vi "tcp发送-main.vi"(0 "服务器网络地址":string="127.0.0.1", 5 "原文件路径（使用对话框）":path=path "C:/Users/Administrator.2W964MZOGI5HE3B/Desktop/labview图片/105256rhad11pc5553vz5e.png", 7 "远程端口或服务名称":u16=6314) -> (4 "运行指示灯":bool=TRUE, 6 "已传百分比":string)   [LabVIEW 2016, in "数据传输系统.lvlib" / "自动更新.lvlib" / "TCP文件传输系统.lvlib" / "TCP发送文件.lvlib"]
panel:
  out "数值":i32
  in  "分帧数(兆)":i64=2
  out "已发帧数":i32
  in  "分一包（兆）":i64=40
  out "侦数":i32
  out "在发第几次":i32
  out "共发送次数":string
  out "网络灯":bool
  in  "停止":bool
  out "错误输出 2":errorcluster caption="错误输出"
  out "错误输出":errorcluster
  out "文件名称":string
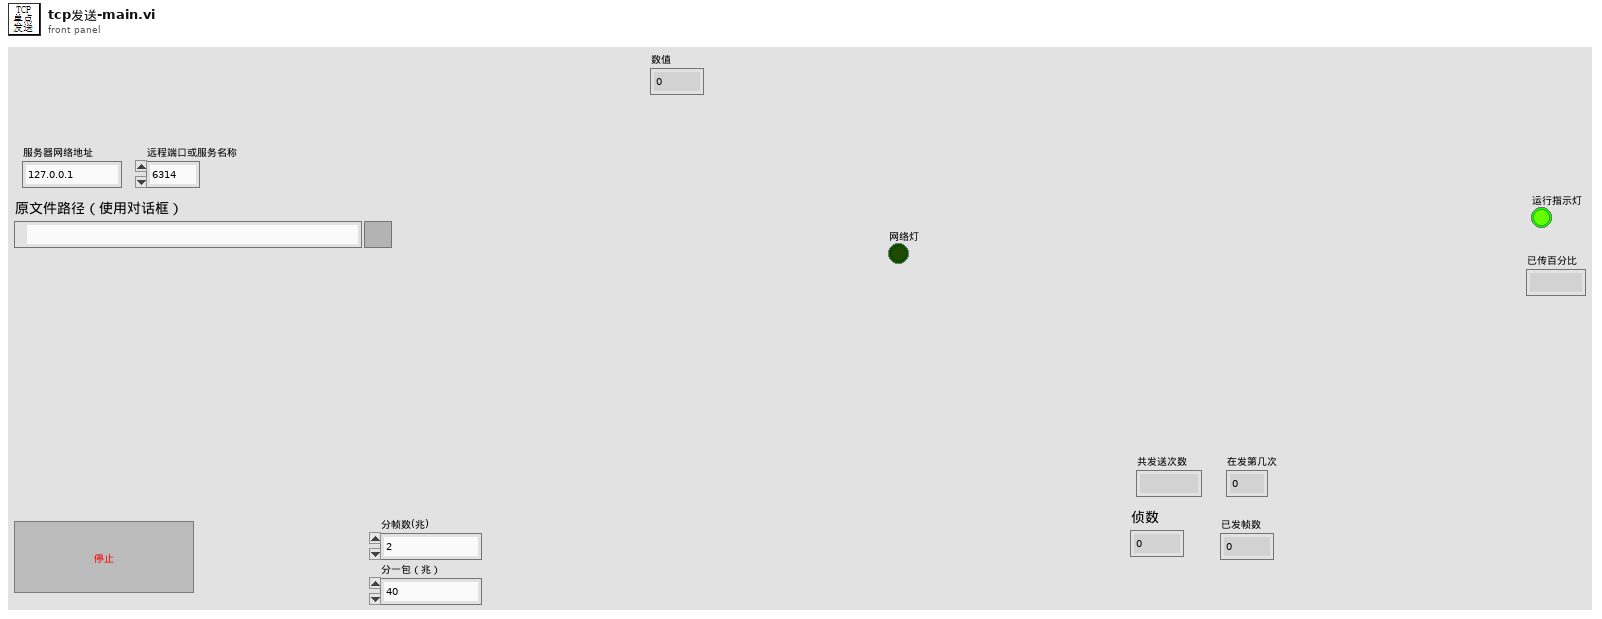
[diagram p1: front panel]
types:
  T1 = enum16{"open", "replace", "create", "open or create", "replace or create", "replace or create with confirmation"}
  T2 = cluster{"网络灯":bool, "发送中":bool, "已发送百分比":u8, "发送成功次数":dbl, "当前步骤":enum16{"readfile", "init", "sendhead", "sendcontent", "sendsuccess", "over"}, "文件名":string, "error out":errorcluster}
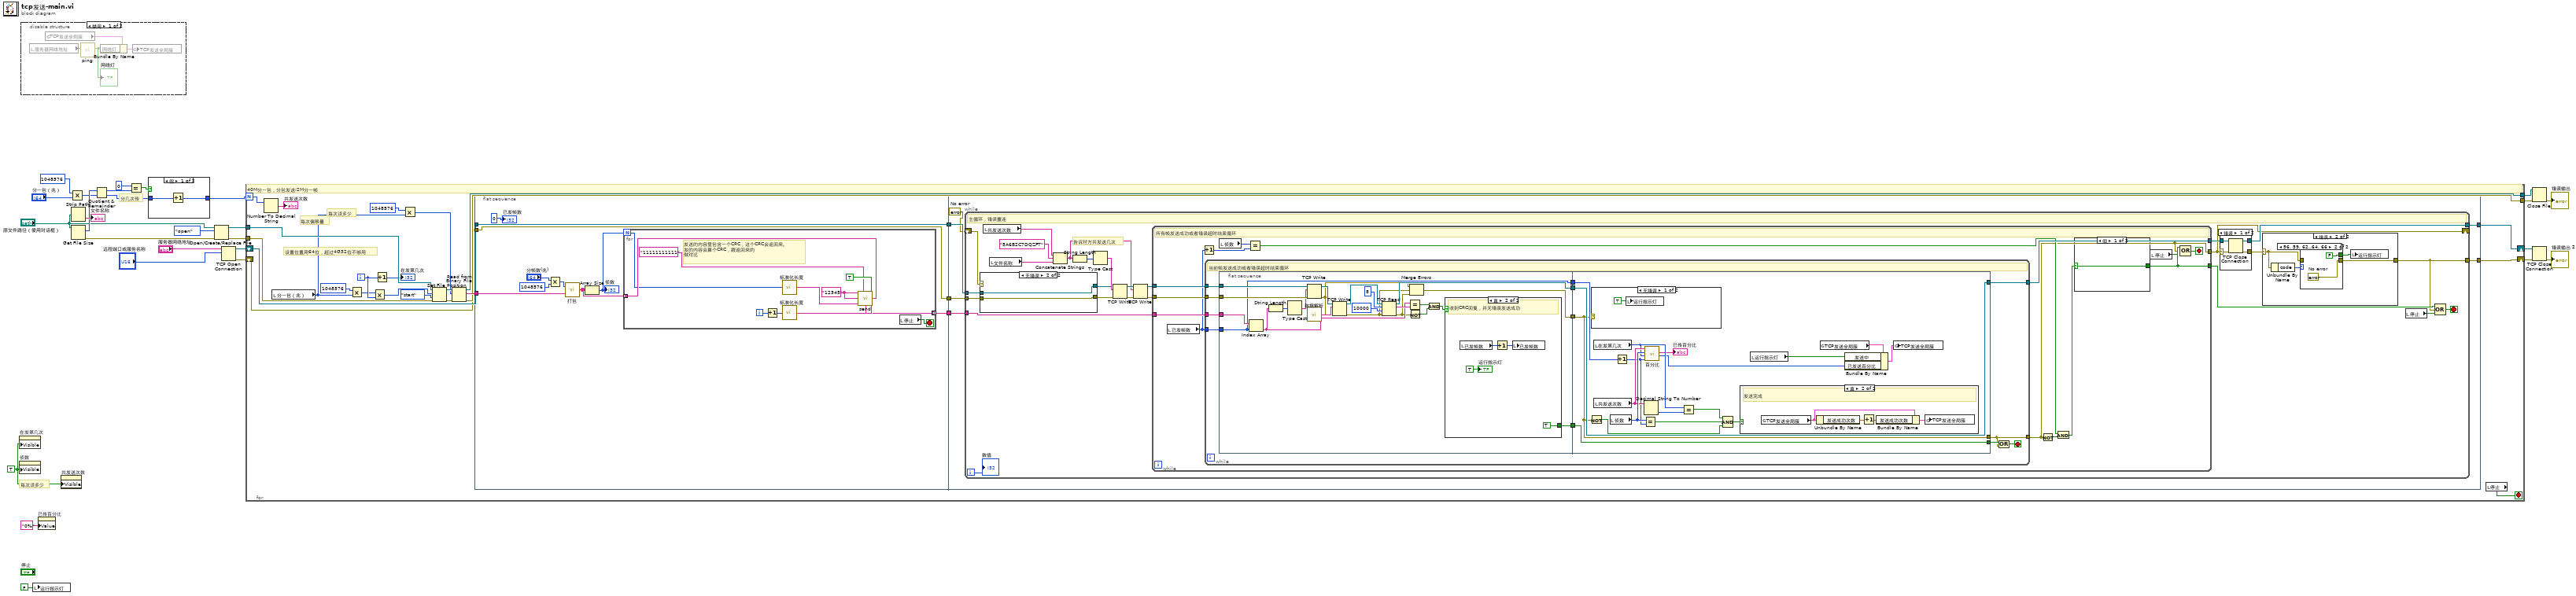
[diagram p0: block diagram]
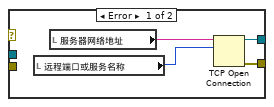
[diagram p5: hidden frame]
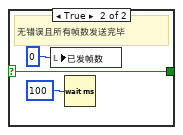
[diagram p6: hidden frame]
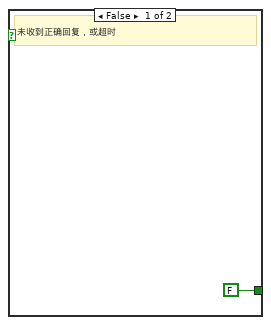
[diagram p7: hidden frame]
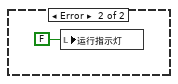
[diagram p8: hidden frame]
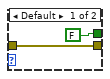
[diagram p11: hidden frame]
diagram:
  w11 = TRUE ("可见")
  # "分几次传"
  # "每次读多少"
  n1 = property on="在发第几次" class="DigNum (严格)"("Visible"=w11) -> ()  [unwired: 2 in, 2 out]
  n2 = property on="侦数" class="DigNum (严格)"("Visible"=w11) -> ()  [unwired: 2 in, 2 out]
  n3 = disable-structure shown="禁用" {
    frame Disabled {
      n4 = local read "服务器网络地址"() -> (w32:string)
      n5 = global read "全局变量1.vi" "TCP发送全局簇"() -> (w30:T2)
      n6 = call "ping.vi"("IP"=w32) -> ("ping结果"=w29:bool)  [unwired: 10 in]
      "网络灯" <- w29
      n7 = Bundle By Name(cluster=w30, "网络灯"=w29) -> (w31:T2)
      n8 = global write "全局变量1.vi" "TCP发送全局簇"(w31) -> ()
    }
    frame Enabled {
    }
  }
  n9 = local write "运行指示灯"(FALSE ("运行指示灯")) -> ()
  n10 = property on="已传百分比" class="Str"("Value"="0%" ("已传百分比")) -> ()  [unwired: 2 in, 2 out]
  n11 = property on="共发送次数" class="Str"("Visible"=w11) -> ()  [unwired: 2 in, 2 out]
  n12 = Multiply(x=i64 1048576 ("y"), y="分一包（兆）") -> (x*y=w3:i64)
  n13 = Strip Path(path="原文件路径（使用对话框）") -> (name=→"文件名称":string)  [unwired: 1 out]
  n14 = Get File Size(file="原文件路径（使用对话框）") -> (size (in bytes)=w9:i64, 0:w10:errorcluster)  [unwired: 1 in, 1 out]
  n15 = Quotient & Remainder(x=w9, y=w3) -> (x-y*floor(x/y)=w25:i64, floor(x/y)=w21:i64)
  n16 = Equal?(x=0, y=w25) -> (x = y?=w23:bool)
  n17 = case shown="假" w23 {
    tunnel: [w33 w35] -> w22
    tunnel: w21 -> [w34 w35]
    frame False {
      n18 = Increment(x=w34) -> (x+1=w33:i64)
    }
    frame True {
    }
  }
  n19 = Open/Create/Replace File(file path (use dialog)="原文件路径（使用对话框）", error in=w10, operation (0:open)=T1."open" ("操作(0:open)")) -> (refnum out=w7:refnum<file>, error out=w6:errorcluster)  [unwired: 3 in, 1 out]
  n20 = TCP Open Connection(address="服务器网络地址", remote port or service name="远程端口或服务名称") -> (connection ID=w13:refnum<k5>, error out=w12:errorcluster)  [unwired: 3 in]
  n21 = for {
    N: w22 -> [w42]
    tunnel: w6 -> [w57]
    tunnel: w7 -> [w56]
    tunnel: [w52] -> w19
    tunnel: [w51] -> w20
    shift-right: [w46] -> w15
    shift-left: w13 -> [w45]
    shift-right: [w47] -> w16
    shift-left: w12 -> [w44]
    i -> [w50]
    stop <- w36 stop-if-true
    # "设置位置用64位，超过4G32位不够用"
    # "每次读多少"
    # "每次偏移量"
    # "40M分一包，分包发送;2M分一帧"
    n22 = Number To Decimal String(number=w42) -> (decimal integer string=→"共发送次数":string)  [unwired: 1 in]
    n23 = local read "分一包（兆）"() -> (w38:i64)
    n24 = Multiply(x=i64 1048576 ("偏移量（字节）（0）"), y=w38) -> (x*y=w40:i64)
    n25 = Multiply(x=w40, y=w50) -> (x*y=w58:i64)
    n26 = Increment(x=w50) -> (x+1=→"在发第几次":i32)
    n27 = Multiply(x=1048576 ("总数(1)"), y=w38) -> (x*y=w37:i64)
    n28 = Set File Position(offset (in bytes) (0)=w58, refnum=w56, from (0:start)=enum16{"start", "end", "current"}."start" ("自（0:起始）"), error in=w57) -> (refnum out=w60:refnum<file>, error out=w61:errorcluster)
    n29 = Read from Binary File(8:w61, 10:w37, 11:w60) -> (0:w52:errorcluster, 2:w55:string, 3:w51:refnum<file>)  [unwired: 3 in, 1 out]
    n30 = flat-sequence {
      tunnel: w55 -> [w66]
      tunnel: [w69] -> w53
      tunnel: [w68] -> w49
      tunnel: w45 -> [w68]
      tunnel: [w67] -> w48
      tunnel: w44 -> [w67]
      tunnel: w53 -> [w88]
      tunnel: w49 -> [w87]
      tunnel: w48 -> [w86]
      tunnel: [w85] -> w47
      tunnel: [w84] -> w46
      frame #0 {
        n31 = Multiply(x="分帧数(兆)", y=i64 1048576) -> (x*y=w65:i64)
        n32 = call "打包.vi"("总内容"=w66, "分包大小"=w65) -> ("分包数组"=w64:string[])
        n33 = Array Size(array=w64) -> (size(s)=w71:i32)
        "侦数" <- w71
        n34 = for {
          N: w71 -> [w77]
          tunnel: w64 -> [w82] mode=indexing
          tunnel: [w75] -> w69 mode=indexing
          i -> [w81]
          stop <- w72 stop-if-true
          w74 = "12345" ("内容说明（文件名）")
          # "发送的内容里包含一个CRC，这个CRC会返回来。\n发的内容会算个CRC，跟返回来的\n做对比"
          n35 = Increment(x=w81) -> (x+1=w76:i32)
          n36 = call "标准化长度.vi"("原长度"=w77) -> ("标准化长度"=w80:string)
          n37 = call "标准化长度.vi"("原长度"=w76) -> ("标准化长度"=w79:string)
          n38 = call "send.vi"("内容标识"=w74, "时标"="11111111111", "发送"=TRUE, "内容说明（文件名）"=w74, "帧内容"=w82, "帧数"=w80, "帧号"=w79) -> ("连接的字符串"=w75:string)  [unwired: 6 in, 2 out]
          n39 = local read "停止"() -> (w72:bool)
        }
        "已发帧数" <- 0 ("数值")
      }
      frame #1 {
        w83 = errorcluster {"status"=FALSE, "code"=0, "source"=""}  # No error
        n40 = while {
          tunnel: w88 -> [w99]
          tunnel: w87 -> [w98]
          tunnel: w86 -> [w97]
          tunnel: [w96] -> w85
          tunnel: [w95] -> w84
          shift-right: [w94] -> _
          shift-left: w83 -> [w93]
          i -> [w89]
          stop <- w111 stop-if-true
          # "告诉对方共发送几次"
          # "主循环，错误重连"
          n41 = case shown="无错误" w93 {
            tunnel: [w123 w125] -> w92
            tunnel: w98 -> [_ w125]
            tunnel: [w122 w124] -> w91
            tunnel: w97 -> [_ w124]
            frame Error {
              n42 = local read "远程端口或服务名称"() -> (w120:u16)
              n43 = local read "服务器网络地址"() -> (w121:string)
              n44 = TCP Open Connection(address=w121, remote port or service name=w120) -> (connection ID=w123:refnum<k5>, error out=w122:errorcluster)  [unwired: 3 in]
            }
            frame No Error {
            }
          }
          n45 = local read "共发送次数"() -> (w102:string)
          n46 = local read "文件名称"() -> (w103:string)
          n47 = Concatenate Strings(w102, "5A6B2C7DQZFT" ("字符串"), w103) -> (w100:string)
          n48 = String Length(string=w100) -> (length=w109:i32)
          n49 = Type Cast(x=w109) -> (*(type *) &x=w108:string)  [unwired: 1 out]
          n50 = TCP Write(connection ID=w92, data in=w108, error in (no error)=w91) -> (connection ID out=w106:refnum<k5>, error out=w107:errorcluster)  [unwired: 2 out]
          n51 = TCP Write(connection ID=w106, data in=w100, error in (no error)=w107) -> (connection ID out=w105:refnum<k5>, error out=w104:errorcluster)  [unwired: 2 out]
          n52 = while {
            tunnel: w105 -> [w139]
            tunnel: w104 -> [w137]
            tunnel: [w128] -> w94
            tunnel: [w135] -> w113
            tunnel: [w133] -> w110
            tunnel: w99 -> [w134]
            stop <- w138 stop-if-true
            # "所有帧发送成功或者错误超时结束循环"
            n53 = local read "已发帧数"() -> (w132:i32)
            n54 = Increment(x=w132) -> (x+1=w131:i32)
            n55 = while {
              tunnel: w132 -> [w154]
              tunnel: w134 -> [w152]
              tunnel: w139 -> [w155]
              tunnel: [w151] -> w135
              tunnel: w137 -> [w153]
              tunnel: [w149] -> w128
              stop <- w148 stop-if-true
              # "当前帧发送成功或者错误超时结束循环"
              n56 = flat-sequence {
                tunnel: w155 -> [w176]
                tunnel: w154 -> [w163]
                tunnel: w153 -> [w175]
                tunnel: w152 -> [w172]
                tunnel: [w170] -> w147
                tunnel: [w169] -> w146
                tunnel: [w156] -> w145
                tunnel: [w163] -> w144
                tunnel: [w189] -> w149
                tunnel: [w200] -> w150
                tunnel: [w201] -> w151
                tunnel: w147 -> [w201]
                tunnel: w146 -> [w200]
                tunnel: w145 -> [w189]
                tunnel: w144 -> [w192]
                frame #0 {
                  n57 = Index Array(array=w172, index=w163) -> (element=w168:string)
                  n58 = String Length(string=w168) -> (length=w177:i32)
                  n59 = Type Cast(x=w177) -> (*(type *) &x=w171:string)  [unwired: 1 out]
                  n60 = TCP Write(connection ID=w176, data in=w171, error in (no error)=w175) -> (connection ID out=w178:refnum<k5>, error out=w158:errorcluster)  [unwired: 2 out]
                  n61 = call "数据解析.vi"("data in"=w168) -> ("data out"=w167:string, "CRC"=w165:string)  [unwired: 4 in, 9 out]
                  n62 = TCP Write(connection ID=w178, data in=w167, error in (no error)=w158) -> (connection ID out=w174:refnum<k5>, error out=w157:errorcluster)  [unwired: 2 out]
                  n63 = TCP Read(connection ID=w174, bytes to read=8 ("读取的字节"), error in (no error)=w157, 9:10000 ("超时毫秒(25000)")) -> (connection ID out=w170:refnum<k5>, data out=w166:string, error out=w159:errorcluster)  [unwired: 1 in]
                  n64 = Equal?(x=w165, y=w166) -> (x = y?=w162:bool)
                  n65 = Not(x=w159) -> (.not. x?=w161:bool)
                  n66 = Merge Errors(w158, w157, w159) -> (w156:errorcluster)
                  n67 = And(x=w162, y=w161) -> (x .and. y?=w160:bool)
                  n68 = case shown="真" w160 {
                    tunnel: [FALSE TRUE] -> w169
                    frame False {
                      # "未收到正确回复，或超时"
                    }
                    frame True {
                      # "收到CRC回复，并无错误发送成功"
                      n69 = local read "已发帧数"() -> (w182:i32)
                      n70 = Increment(x=w182) -> (x+1=w183:i32)
                      n71 = local write "已发帧数"(w183) -> ()
                      "运行指示灯" <- TRUE
                    }
                  }
                }
                frame #1 {
                  n72 = Not(x=w189) -> (.not. x?=w190:bool)
                  n73 = case shown="无错误" w189 {
                    frame No Error {
                      n74 = local write "运行指示灯"(TRUE ("运行指示灯")) -> ()
                    }
                    frame Error {
                      n75 = local write "运行指示灯"(FALSE ("运行指示灯")) -> ()
                    }
                  }
                  n76 = local read "在发第几次"() -> (w196:i32)
                  n77 = local read "共发送次数"() -> (w198:string)
                  n78 = local read "侦数"() -> (w199:i32)
                  n79 = Increment(x=w192) -> (x+1=w191:i32)
                  n80 = Equal?(x=w199, y=w191) -> (x = y?=w194:bool)
                  n81 = Decimal String To Number(string=w198) -> (number=w197:i32)  [unwired: 2 in, 1 out]
                  n82 = call "百分比.vi"("已发帧数 2"=w191, "发第几次"=w196, "帧数"=w199, "共发送次数"=w198) -> ("已发送百分比"=w184:u8, "已传百分比"=→"已传百分比":string)  [unwired: 6 in]
                  n83 = Equal?(x=w196, y=w197) -> (x = y?=w195:bool)
                  n84 = Compound Arithmetic op=AND(w195, w194, w190) -> (w193:bool)
                  n85 = case shown="真" w193 {
                    frame False {
                    }
                    frame True {
                      # "发送完成"
                      n86 = global read "全局变量1.vi" "TCP发送全局簇"() -> (w204:T2)
                      n87 = Unbundle By Name(w204) -> ("发送成功次数"=w205:dbl)
                      n88 = Increment(x=w205) -> (x+1=w206:dbl)
                      n89 = Bundle By Name(cluster=w204, "发送成功次数"=w206) -> (w207:T2)
                      n90 = global write "全局变量1.vi" "TCP发送全局簇"(w207) -> ()
                    }
                  }
                  n91 = local read "运行指示灯"() -> (w188:bool)
                  n92 = global read "全局变量1.vi" "TCP发送全局簇"() -> (w186:T2)
                  n93 = Bundle By Name(cluster=w186, "发送中"=w188, "已发送百分比"=w184) -> (w187:T2)
                  n94 = global write "全局变量1.vi" "TCP发送全局簇"(w187) -> ()
                }
              }
              n95 = Compound Arithmetic op=OR(w150, w149) -> (w148:bool)
            }
            n96 = local read "侦数"() -> (w136:i32)
            n97 = Equal?(x=w136, y=w131) -> (x = y?=w130:bool)
            n98 = Not(x=w128) -> (.not. x?=w127:bool)
            n99 = Compound Arithmetic op=AND(w130, w127) -> (w129:bool)
            n100 = case shown="假" w129 {
              selector: w129 -> [w140 w142]
              tunnel: [w140 w142] -> w133
              frame False {
              }
              frame True {
                # "无错误且所有帧数发送完毕"
                n101 = local write "已发帧数"(0 ("已发帧数")) -> ()
                n102 = Wait (ms)(milliseconds to wait=u32 100 ("等待时间（毫秒）")) -> ()  [unwired: 1 out]
              }
            }
            n103 = local read "停止"() -> (w126:bool)
            n104 = Compound Arithmetic op=OR(w133, w128, w126) -> (w138:bool)
          }
          n105 = case shown="错误" w94 {
            selector: w94 -> [w114 w118]
            tunnel: w113 -> [w117 w119]
            tunnel: [w116 w118] -> w112
            tunnel: [w115 w119] -> w95
            frame Error {
              n106 = TCP Close Connection(connection ID=w117, error in (no error)=w114) -> (connection ID out=w115:refnum<k5>, error out=w116:errorcluster)  [unwired: 1 in]
            }
            frame No Error {
            }
          }
          n107 = case shown="错误" w112 {
            selector: w112 -> [w208 w211]
            tunnel: [w208 w210] -> w96
            frame No Error {
            }
            frame Error {
              n108 = Unbundle By Name(w211) -> ("code"=w212:i32)
              n109 = case shown="56, 59, 62..64, 66" w212 {
                tunnel: w211 -> [w214 _]
                tunnel: [w214 w216] -> w210
                tunnel: [FALSE FALSE] -> w209
                frame Default {
                }
                frame 56, 59, 62..64, 66 {
                  w216 = errorcluster {"status"=FALSE, "code"=0, "source"=""}  # No error
                }
              }
              n110 = local write "运行指示灯"(w209) -> ()
            }
          }
          n111 = local read "停止"() -> (w90:bool)
          n112 = Compound Arithmetic op=OR(w110, w96, w90) -> (w111:bool)
          "数值" <- w89
        }
      }
    }
    n113 = local read "停止"() -> (w36:bool)
  }
  n114 = Close File(refnum=w20, error in=w19) -> (error out=→"错误输出":errorcluster)  [unwired: 1 out]
  n115 = TCP Close Connection(connection ID=w15, error in (no error)=w16) -> (error out=→"错误输出 2":errorcluster)  [unwired: 1 in, 1 out]
